vi "TimeGatedImageGlobal.vi"(0 "error in":errorcluster, 3 "RGB / False":enum16{"RGB", "False color"}(ring), 4 "add string":string, 5 "threshold":cluster{"max":u32, "min":u32}, 6 "input":u32[][][][](array[numeric]), 7 "router channel":u16, 8 "action":T1(ring), 9 "title":string) -> (1 "title out":string, 2 "Image Duplicate (out)":T2)   [LabVIEW 2009]
uses:
  <vilib>/vision/Image Controls.llb/IMAQ Image.ctl
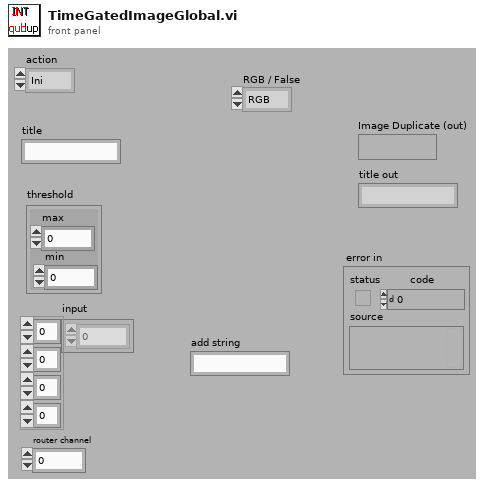
[diagram p1: front panel]
types:
  T1 = enum16{"Ini", "Get", "Set", "Refresh", "dump", "move", "name"}
  T2 = typedef "IMAQ Image.ctl" = refnum<image>
  T3 = enum16{"Ini", "Get", "Set", "Refresh", "dump", "move"}
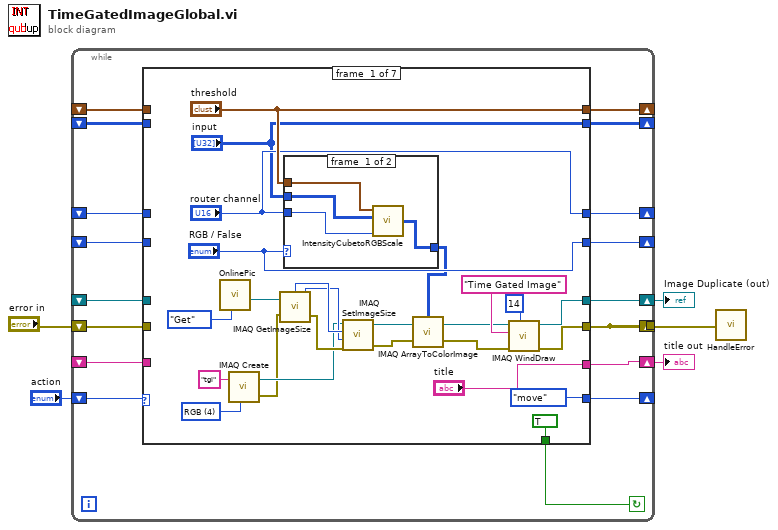
[diagram p0: block diagram]
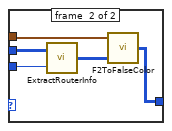
[diagram p2: hidden frame]
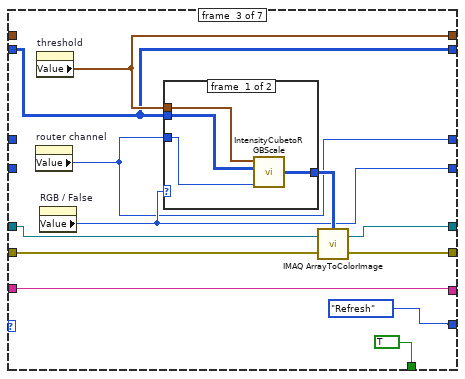
[diagram p4: hidden frame]
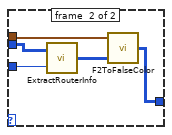
[diagram p5: hidden frame]
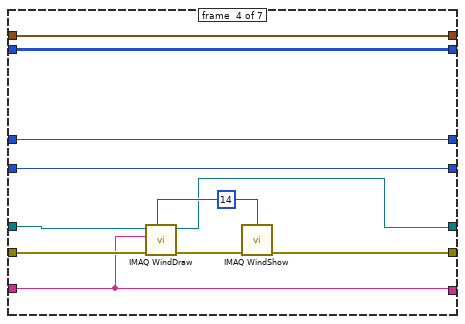
[diagram p6: hidden frame]
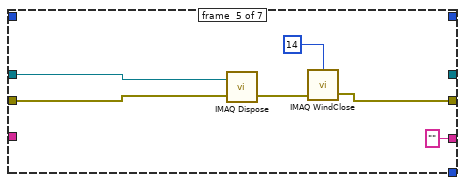
[diagram p7: hidden frame]
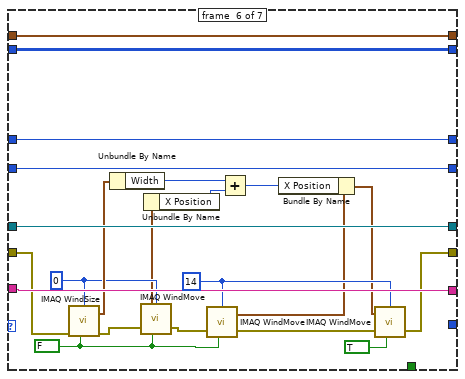
[diagram p8: hidden frame]
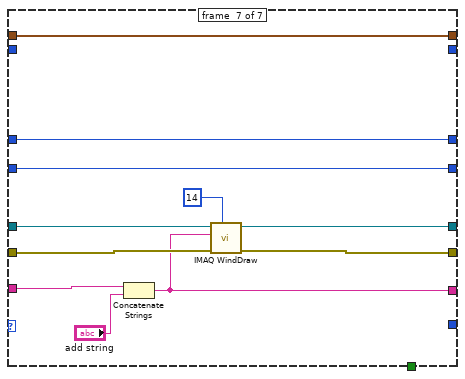
[diagram p9: hidden frame]
diagram:
  n1 = while {
    shift-right: [w22] -> w5
    shift-left: _ -> [w21]
    shift-right: [w16] -> _
    shift-left: "action" -> [w19]
    shift-right: [w17] -> w1
    shift-left: "error in" -> [w18]
    tunnel: [w17] -> _
    shift-right: [w14] -> w3
    shift-left: _ -> [w15]
    shift-right: [w13] -> _
    shift-left: _ -> [w12]
    shift-right: [w11] -> _
    shift-left: _ -> [w10]
    shift-right: [w9] -> _
    shift-left: _ -> [w6]
    shift-right: [w8] -> _
    shift-left: _ -> [w7]
    stop <- w20 continue-if-true
    n2 = case shown="\"Set\"" w19 {
      tunnel: [w42 w62 w70 w89 _ w121 w131] -> w22
      tunnel: [w41 _ w69 w93 w95 w109 w130] -> w17
      tunnel: w21 -> [_ w62 w71 w90 w98 w121 w132]
      tunnel: [TRUE _ TRUE _ _ _ _] -> w20
      tunnel: w18 -> [_ _ w68 w92 w99 w120 w133]
      tunnel: [T3."move" ("Enum") _ enum16{"Ini", "Get", "Set", "Refresh"}."Refresh" ("Enum") _ _ _ _] -> w16
      tunnel: w15 -> [_ w61 w72 w88 _ w122 w126]
      tunnel: ["title" w61 w72 w88 "" ("title") w122 w128] -> w14
      tunnel: ["threshold" w60 w67 w87 _ w104 w125] -> w13
      tunnel: w12 -> [_ w60 _ w87 _ w104 w125]
      tunnel: ["input" w59 w63 w86 _ w103 _] -> w11
      tunnel: w10 -> [_ w59 w63 w86 _ w103 _]
      tunnel: ["RGB / False" w57 w65 w84 _ w101 w124] -> w9
      tunnel: ["router channel" w58 w64 w85 _ w102 w123] -> w8
      tunnel: w7 -> [_ w58 _ w85 _ w102 w123]
      tunnel: w6 -> [_ w57 _ w84 _ w101 w124]
      frame #0 {
        w44 = u32 4 items=["8 bits", "16 bits", "Float", "Complex", "RGB", "HSL"] ("Image Type")
        n3 = call "OnlinePic.vi"("action"=enum16{"Get", "Set", "Change", "ini"}."Get" ("Enum")) -> ("Image Out (duplicate)"=w34:T2)  [unwired: 6 in, 4 out]
        n4 = call "IMAQ Create"("Image Name"="tgi", "Image Type"=w44) -> ("New Image"=w33:T2, "error out"=w32:errorcluster)  [unwired: 3 in]
        n5 = call "IMAQ GetImageSize"("Image"=w34, "error in (no error)"=w32) -> ("Y Resolution"=w36:i32, "X Resolution"=w37:i32, "error out"=w35:errorcluster)  [unwired: 2 in]
        n6 = case shown="\"RGB\", Default" "RGB / False" {
          tunnel: "threshold" -> [w51 w52]
          tunnel: "input" -> [w50 w55]
          tunnel: [w49 w56] -> w24
          tunnel: "router channel" -> [w48 w53]
          frame #0 {
            n7 = call "IntensityCubetoRGBScale.vi"("Router"=w48, "Trace"=w50, "threshold"=w51) -> ("RGB Scale"=w49:u32[][])  [unwired: 1 in]
          }
          frame #1 {
            n8 = call "ExtractRouterInfo.vi"("router channel"=w53, "Array 2"=w55) -> ("Array"=w54:u32[][][][])
            n9 = call "F2ToFalseColor.vi"("Intensity"=w54, "Threshold (max)"=w52) -> ("FalseColor"=w56:u32[][])  [unwired: 1 in]
          }
        }
        n10 = call "IMAQ SetImageSize"("error in (no error)"=w35, "Y Resolution"=w36, "X Resolution"=w37, "Image"=w33) -> ("error out"=w30:errorcluster, "Image Out"=w31:T2)  [unwired: 1 in]
        n11 = call "IMAQ ArrayToColorImage"("Image Pixels (U32)"=w24, "Image"=w31, "error in (no error)"=w30) -> ("Image Out"=w28:T2, "error out"=w29:errorcluster)  [unwired: 2 in]
        n12 = call "IMAQ WindDraw"("Window Number (0...15)"=14, "error in (no error)"=w29, "Title"="Time Gated Image", "Image"=w28) -> ("error out"=w41:errorcluster, "Image Out (duplicate)"=w42:T2)  [unwired: 6 in]
      }
      frame #1 {
      }
      frame #2 {
        n13 = property on="router channel" class="Digital (strict)"() -> ("Value"=w64:u16)  [unwired: 2 in, 2 out]
        n14 = property on="threshold" class="Cluster (strict)"() -> ("Value"=w67:cluster{"max":u32, "min":u32})  [unwired: 2 in, 2 out]
        n15 = property on="RGB / False" class="Enum (strict)"() -> ("Value"=w65:enum16{"RGB", "False color"})  [unwired: 2 in, 2 out]
        n16 = case shown="\"False color\"" w65 {
          tunnel: w67 -> [w78 w79]
          tunnel: w63 -> [w77 w82]
          tunnel: [w76 w83] -> w66
          tunnel: w64 -> [w75 w80]
          frame #0 {
            n17 = call "IntensityCubetoRGBScale.vi"("Router"=w75, "Trace"=w77, "threshold"=w78) -> ("RGB Scale"=w76:u32[][])  [unwired: 1 in]
          }
          frame #1 {
            n18 = call "ExtractRouterInfo.vi"("router channel"=w80, "Array 2"=w82) -> ("Array"=w81:u32[][][][])
            n19 = call "F2ToFalseColor.vi"("Intensity"=w81, "Threshold (max)"=w79) -> ("FalseColor"=w83:u32[][])  [unwired: 1 in]
          }
        }
        n20 = call "IMAQ ArrayToColorImage"("Image Pixels (U32)"=w66, "Image"=w71, "error in (no error)"=w68) -> ("Image Out"=w70:T2, "error out"=w69:errorcluster)  [unwired: 2 in]
      }
      frame #3 {
        w94 = 14 ("Window Number (0...15)")
        n21 = call "IMAQ WindDraw"("Window Number (0...15)"=w94, "error in (no error)"=w92, "Title"=w88, "Image"=w90) -> ("error out"=w91:errorcluster, "Image Out (duplicate)"=w89:T2)  [unwired: 6 in]
        n22 = call "IMAQ WindShow"("error in (no error)"=w91, "Window Number (0...15)"=w94) -> ("error out"=w93:errorcluster)  [unwired: 4 in, 2 out]
      }
      frame #4 {
        n23 = call "IMAQ Dispose"("Image"=w98, "error in (no error)"=w99) -> ("error out"=w97:errorcluster)  [unwired: 4 in]
        n24 = call "IMAQ WindClose"("Window Number (0...15)"=14, "error in (no error)"=w97) -> ("error out"=w95:errorcluster)  [unwired: 4 in]
      }
      frame #5 {
        w114 = FALSE ("Get/Set Status? (Set)")
        w112 = 14 ("Window Number (0...15)")
        w117 = 0 ("Window Number")
        n25 = call "IMAQ WindSize"("error in (no error)"=w120, "Get/Set Status? (Set)"=w114, "Window Number"=w117) -> ("error out"=w119:errorcluster, "Width & Height out"=w118:cluster{"Width":i32, "Height":i32})  [unwired: 3 in, 1 out]
        n26 = Unbundle By Name(w118) -> ("Width"=w106:i32)
        n27 = call "IMAQ WindMove"("Window Number (0...15)"=w117, "Get/Set Status? (Set)"=w114, "error in (no error)"=w119) -> ("Coordinates (screen)"=w108:cluster{"X Position":i32, "Y Position":i32}, "error out"=w116:errorcluster)  [unwired: 2 in]
        n28 = Unbundle By Name(w108) -> ("X Position"=w107:i32)
        n29 = call "IMAQ WindMove"("Window Number (0...15)"=w112, "Get/Set Status? (Set)"=w114, "error in (no error)"=w116) -> ("Coordinates (screen)"=w111:cluster{"X Position":i32, "Y Position":i32}, "error out"=w115:errorcluster)  [unwired: 2 in]
        n30 = Add(x=w106, y=w107) -> (x+y=w105:i32)
        n31 = Bundle By Name(cluster=w111, "X Position"=w105) -> (w110:cluster{"X Position":i32, "Y Position":i32})
        n32 = call "IMAQ WindMove"("Window Number (0...15)"=w112, "Coordinates (screen)"=w110, "Get/Set Status? (Set)"=TRUE, "error in (no error)"=w115) -> ("error out"=w109:errorcluster)  [unwired: 1 in, 1 out]
      }
      frame #6 {
        n33 = Concatenate Strings(w126, "add string") -> (w128:string)
        n34 = call "IMAQ WindDraw"("Window Number (0...15)"=14, "error in (no error)"=w133, "Title"=w128, "Image"=w132) -> ("error out"=w130:errorcluster, "Image Out (duplicate)"=w131:T2)  [unwired: 6 in]
      }
    }
  }
  "Image Duplicate (out)" <- w5
  "title out" <- w3
  n35 = call "HandleError.vi"("error in (no error)"=w1) -> ()
